vi "Error Processor.vi"(8 "error in (no error)":errorcluster, 11 "Kasli Writer in":refnum<class "Kasli Writer.lvclass">) -> (0 "error out":errorcluster, 3 "Kasli Writer out":refnum<class "Kasli Writer.lvclass">)   [LabVIEW 2020, in "TALOS.lvlib" / "Kasli Listener and Writer.lvlib" / "Kasli Writer.lvclass"]
doc: "Use this VI to process all the error that are solvable inside this specific uService. Whatever is not possible to process, let it leave this VI and it will be processed by the Error Manager of the Distributed System."
uses:
  Kasli Writer.lvclass
  System uServices/TCP Writer/TCP Writer/TCP Writer.lvclass
  Kasli Writer.lvclass/Kasli Writer.ctl
  TALOS.lvlib
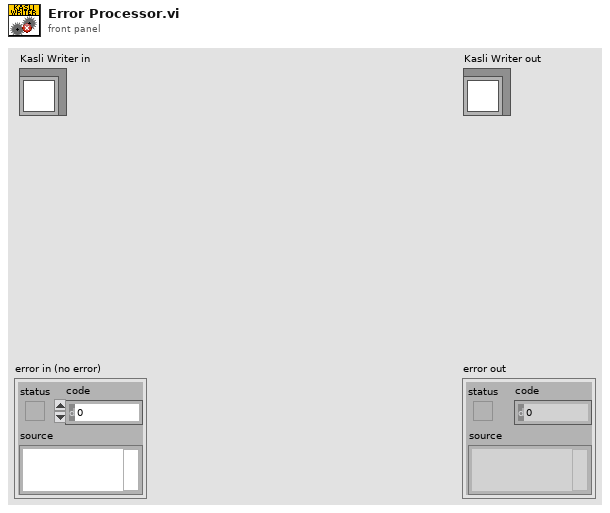
[diagram p1: front panel]
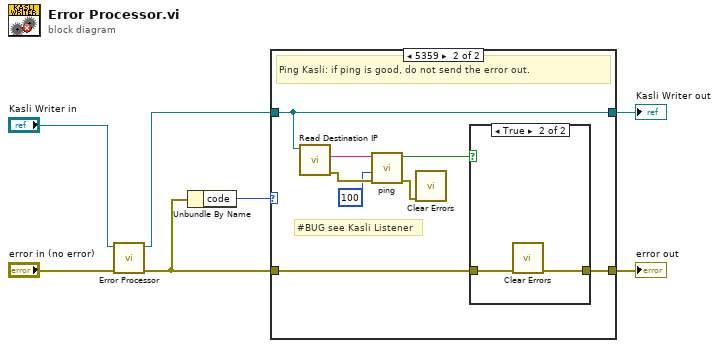
[diagram p0: block diagram]
diagram:
  n1 = call-parent "Error Processor.vi"("error in (no error)"="error in (no error)", "TCP Writer in"="Kasli Writer in") -> ("error out"=w4:errorcluster, "TCP Writer out"=w1:refnum<class "Kasli Writer.lvclass">)  [unwired: 8 in]
  n2 = Unbundle By Name(w4) -> ("code"=w5:i32)
  n3 = case shown="5359" w5 {
    tunnel: [w9 w17] -> w2
    tunnel: w1 -> [w9 w17]
    tunnel: w4 -> [w8 w11]
    tunnel: [w8 w10] -> w3
    frame Default {
      # "Let it through."
    }
    frame 5359 {
      # "#BUG see Kasli Listener"
      # "Ping Kasli: if ping is good, do not send the error out."
      n4 = call-dynamic "Read Destination IP.vi"("TCP Writer in"=w17) -> ("error out"=w15:errorcluster, "Destination IP"=w16:string)  [unwired: 8 in, 1 out]
      n5 = call "ping.vi"("error in (no error)"=w15, "timeout (ms)"=100, "IP/Address"=w16) -> ("error out"=w13:errorcluster, "Success?"=w12:bool)  [unwired: 5 in, 2 out]
      n6 = call <vilib>:"Clear Errors.vi"("error in (no error)"=w13) -> ()  [unwired: 5 in, 2 out]
      n7 = case shown="True" w12 {
        tunnel: w11 -> [w18 w20]
        tunnel: [w18 w19] -> w10
        frame False {
        }
        frame True {
          n8 = call <vilib>:"Clear Errors.vi"("error in (no error)"=w20) -> ("error out"=w19:errorcluster)  [unwired: 5 in, 1 out]
        }
      }
    }
  }
  "error out" <- w3
  "Kasli Writer out" <- w2
